vi "SSR-Test.vi"() -> ()   [LabVIEW 2025]
uses:
  <vilib>/Instr/_visa.llb/VISA Configure Serial Port (Instr).vi
panel:
  in  "Stop":bool
  out "String":string
  in  "Com Port":refnum<visa-resource-name>
  in  "SSR 1":bool
  in  "100 Ohm Load":bool
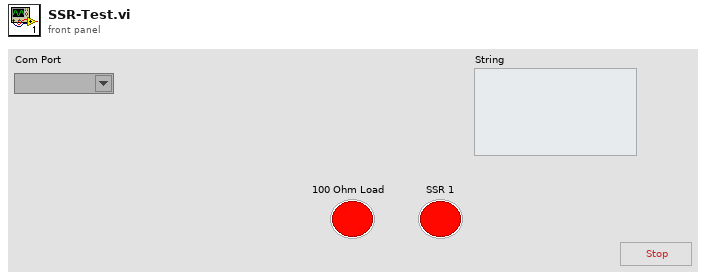
[diagram p1: front panel]
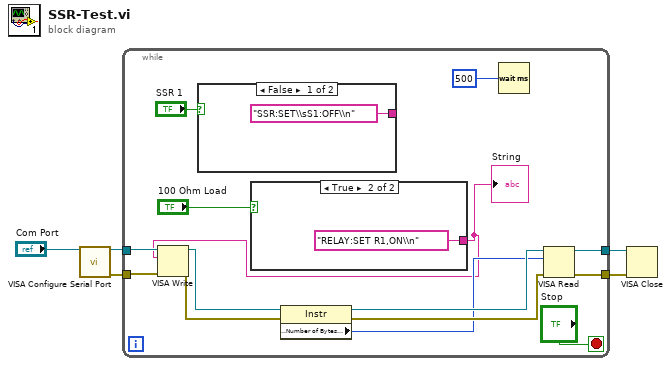
[diagram p0: block diagram]
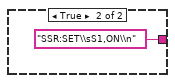
[diagram p2: hidden frame]
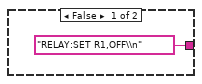
[diagram p3: hidden frame]
diagram:
  n1 = call-poly "VISA Configure Serial Port"("VISA resource name"="Com Port") -> ("VISA resource name out"=w5:refnum<visa-resource-name>, "error out"=w4:errorcluster)  [unwired: 13 in]
  n2 = while {
    tunnel: w5 -> [w14]
    tunnel: [w16] -> w1
    tunnel: w4 -> [w13]
    tunnel: [w17] -> w2
    stop <- "Stop" stop-if-true
    n3 = case shown="False" "SSR 1" {
      tunnel: ["SSR:SET\\sS1:OFF\\n" "SSR:SET\\sS1,ON\\n"] -> _
      frame False {
      }
      frame True {
      }
    }
    n4 = case shown="True" "100 Ohm Load" {
      tunnel: ["RELAY:SET R1,OFF\\n" "RELAY:SET R1,ON\\n"] -> w7
      frame False {
      }
      frame True {
      }
    }
    "String" <- w7
    n5 = VISA Write(VISA resource name=w14, write buffer=w7, error in (no error)=w13) -> (VISA resource name out=w12:refnum<visa-resource-name>, error out=w11:errorcluster)  [unwired: 1 out]
    n6 = property class="Instr"(reference=w12, error in=w11) -> (reference out=w10:refnum<visa-resource-name>, error out=w9:errorcluster, "Serial Settings:Number of Bytes at Serial Port"=w8:u32)
    n7 = Wait (ms)(milliseconds to wait=u32 500) -> ()  [unwired: 1 out]
    n8 = VISA Read(VISA resource name=w10, byte count=w8, error in (no error)=w9) -> (VISA resource name out=w16:refnum<visa-resource-name>, error out=w17:errorcluster)  [unwired: 2 out]
  }
  n9 = VISA Close(VISA resource name=w1, error in (no error)=w2) -> ()  [unwired: 1 out]
